vi "GetDirection.vi"(8 "error in (no error)":errorcluster, 11 "Snake in":refnum<class "Snake.lvclass">) -> (0 "error out":errorcluster, 3 "Snake out":refnum<class "Snake.lvclass">)   [LabVIEW 2019, in "RT_Game.lvlib" / "Snake.lvclass"]
uses:
  Snake.lvclass
  C:/Users/FreshBob/Dropbox/VIs/myRIO_GameConsole/RT/RT_Game/Game/Game.lvclass
  Game/Game.lvclass/Game.ctl
  Snake.lvclass/Snake.ctl
  Game/Game.lvclass
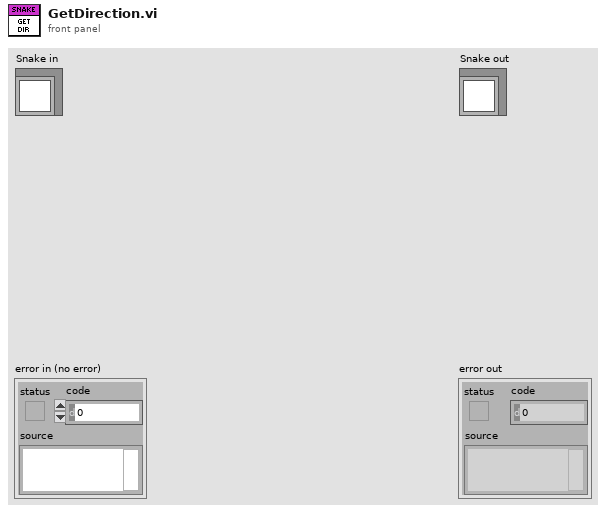
[diagram p1: front panel]
types:
  T1 = cluster{"Controls_1":cluster{"DirectionX":i8, "DirectionY":i8, "Button1":bool, "Button2":bool}, "Controls_2":cluster{"DirectionX":i8, "DirectionY":i8, "Button1":bool, "Button2":bool}, "SystemButton":bool}
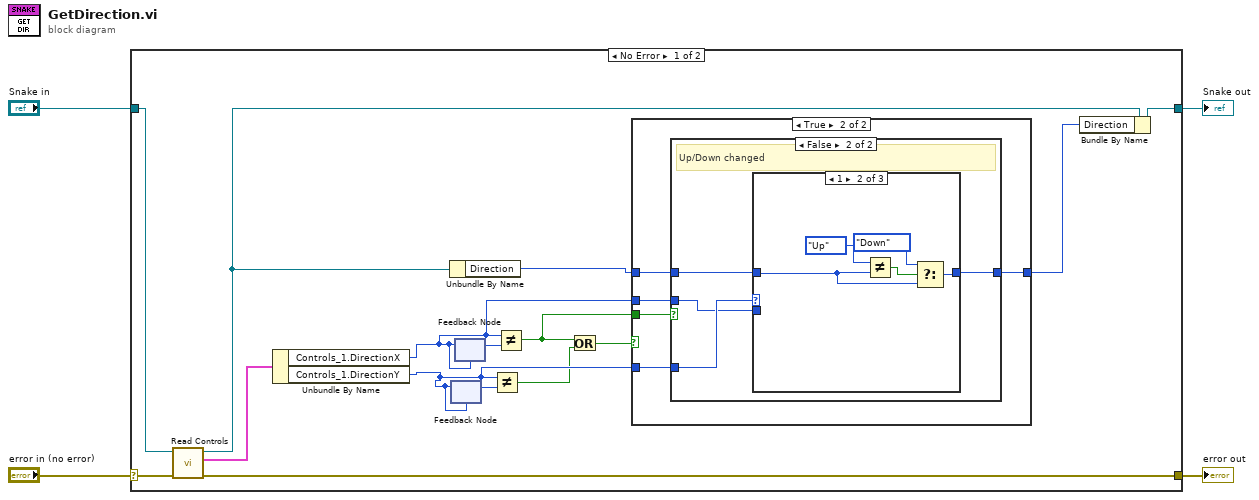
[diagram p0: block diagram]
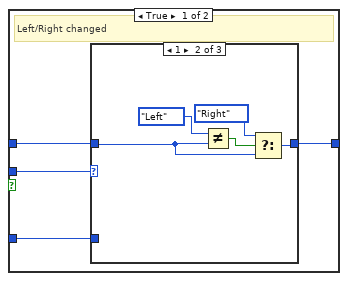
[diagram p3: hidden frame]
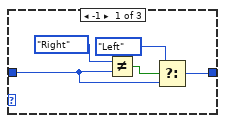
[diagram p4: hidden frame]
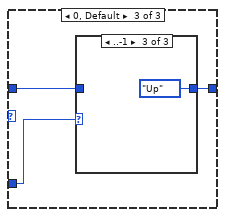
[diagram p5: hidden frame]
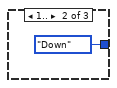
[diagram p7: hidden frame]
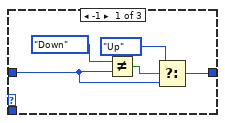
[diagram p8: hidden frame]
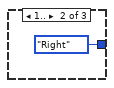
[diagram p10: hidden frame]
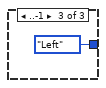
[diagram p11: hidden frame]
diagram:
  n1 = case shown="No Error" "error in (no error)" {
    selector: "error in (no error)" -> [w19 w67]
    tunnel: [w18 w67] -> w3
    tunnel: [w8 w66] -> w1
    tunnel: "Snake in" -> [w17 w66]
    frame No Error {
      n2 = call "Read Controls.vi"("error in (no error)"=w19, "Game in"=w17) -> ("error out"=w18:errorcluster, "Controls"=w16:T1, "Game out"=w6:refnum<class "Snake.lvclass">)  [unwired: 7 in]
      n3 = Unbundle By Name(w16) -> ("Controls_1.DirectionX"=w13:i8, "Controls_1.DirectionY"=w12:i8)
      n4 = Unbundle By Name(w6) -> ("Direction"=w5:enum16{"Up", "Down", "Left", "Right"})
      n5 = feedback #1(w12) -> (w14:i8)
      n6 = feedback-in #1(w12) -> ()
      n7 = feedback-in #2(w13) -> ()
      n8 = feedback #2(w13) -> (w15:i8)
      n9 = Not Equal?(x=w12, y=w14) -> (x != y?=w11:bool)
      n10 = Not Equal?(x=w13, y=w15) -> (x != y?=w9:bool)
      n11 = Or(x=w9, y=w11) -> (x .or. y?=w10:bool)
      n12 = case shown="True" w10 {
        tunnel: w13 -> [_ w24]
        tunnel: w12 -> [_ w21]
        tunnel: w9 -> [_ w25]
        tunnel: w5 -> [w20 w23]
        tunnel: [w20 w22] -> w7
        frame False {
        }
        frame True {
          n13 = case shown="False" w25 {
            tunnel: w24 -> [w29 w46]
            tunnel: w23 -> [w28 w49]
            tunnel: [w27 w48] -> w22
            tunnel: w21 -> [w26 w47]
            frame True {
              # "Left/Right changed"
              n14 = case shown="1" w29 {
                tunnel: [w32 w35 w41] -> w27
                tunnel: w28 -> [w33 w36 w40]
                tunnel: w26 -> [_ _ w42]
                frame -1 {
                  n15 = Not Equal?(x=enum16{"Up", "Down", "Left", "Right"}."Right", y=w33) -> (x != y?=w31:bool)
                  n16 = Select(t=enum16{"Up", "Down", "Left", "Right"}."Left", s=w31, f=w33) -> (s? t:f=w32:enum16{"Up", "Down", "Left", "Right"})
                }
                frame 1 {
                  n17 = Not Equal?(x=enum16{"Up", "Down", "Left", "Right"}."Left", y=w36) -> (x != y?=w39:bool)
                  n18 = Select(t=enum16{"Up", "Down", "Left", "Right"}."Right", s=w39, f=w36) -> (s? t:f=w35:enum16{"Up", "Down", "Left", "Right"})
                }
                frame 0, Default {
                  n19 = case shown="..-1" w42 {
                    tunnel: [w43 enum16{"Up", "Down", "Left", "Right"}."Down" ("Direction") enum16{"Up", "Down", "Left", "Right"}."Up" ("Direction")] -> w41
                    tunnel: w40 -> [w43 _ _]
                    frame 0, Default {
                    }
                    frame 1.. {
                    }
                    frame ..-1 {
                    }
                  }
                }
              }
            }
            frame False {
              # "Up/Down changed"
              n20 = case shown="1" w47 {
                tunnel: [w52 w55 w61] -> w48
                tunnel: w49 -> [w53 w56 w60]
                tunnel: w46 -> [_ _ w62]
                frame -1 {
                  n21 = Not Equal?(x=enum16{"Up", "Down", "Left", "Right"}."Down", y=w53) -> (x != y?=w51:bool)
                  n22 = Select(t=enum16{"Up", "Down", "Left", "Right"}."Up", s=w51, f=w53) -> (s? t:f=w52:enum16{"Up", "Down", "Left", "Right"})
                }
                frame 1 {
                  n23 = Not Equal?(x=enum16{"Up", "Down", "Left", "Right"}."Up", y=w56) -> (x != y?=w59:bool)
                  n24 = Select(t=enum16{"Up", "Down", "Left", "Right"}."Down", s=w59, f=w56) -> (s? t:f=w55:enum16{"Up", "Down", "Left", "Right"})
                }
                frame 0, Default {
                  n25 = case shown="0, Default" w62 {
                    tunnel: [w63 enum16{"Up", "Down", "Left", "Right"}."Right" ("Direction") enum16{"Up", "Down", "Left", "Right"}."Left" ("Direction")] -> w61
                    tunnel: w60 -> [w63 _ _]
                    frame 0, Default {
                    }
                    frame 1.. {
                    }
                    frame ..-1 {
                    }
                  }
                }
              }
            }
          }
        }
      }
      n26 = Bundle By Name(cluster=w6, "Direction"=w7) -> (w8:refnum<class "Snake.lvclass">)
    }
    frame Error {
    }
  }
  "error out" <- w3
  "Snake out" <- w1
